vi "Compare local and remote personalities.vi"(8 "error in (no error)":errorcluster, 10 "DB personality":T1, 11 "roboRIO personality":T1) -> (0 "error out":errorcluster, 3 "Loaded Personality":T1)   [LabVIEW 2018, in "Personalities Tool.lvlib"]
doc: "This VI resolves conflicts between personalities in the roboRIO and in the local DB."
uses:
  Personalities Tool.lvlib
  Controls/Personality Type.ctl
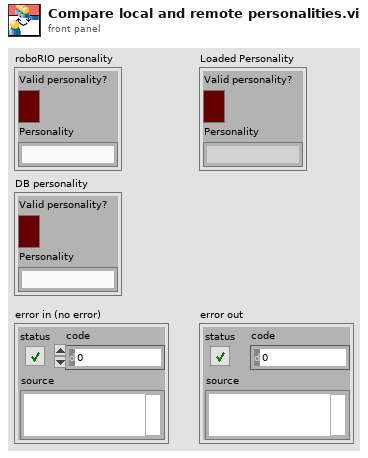
[diagram p1: front panel]
types:
  T1 = typedef "Personalities Tool.lvlib/Personality Type.ctl" = cluster{"Valid personality?":bool, "Personality":string}
  T2 = cluster{"Valid personality?":bool, "Personality":string}
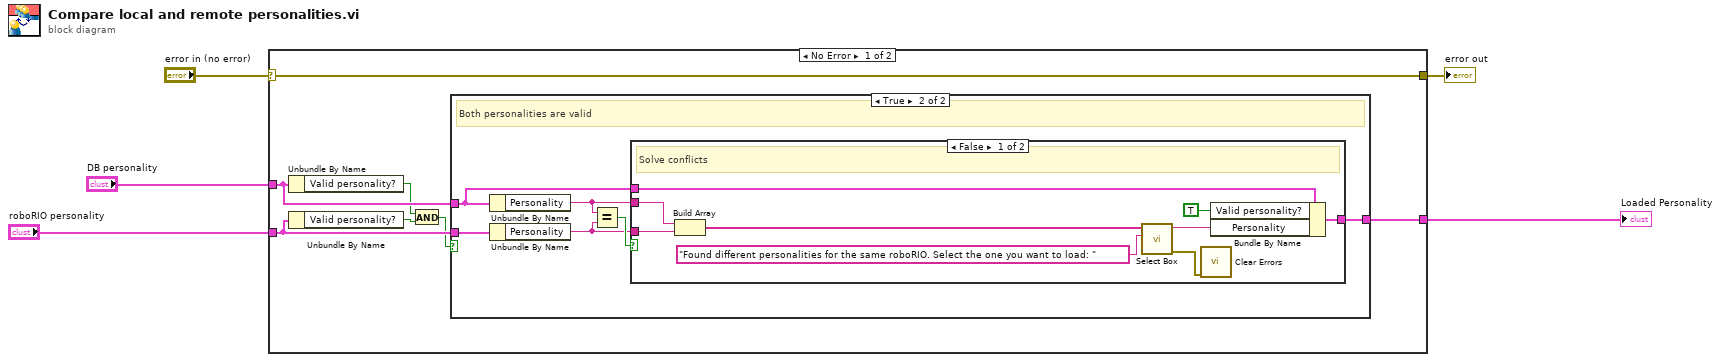
[diagram p0: block diagram]
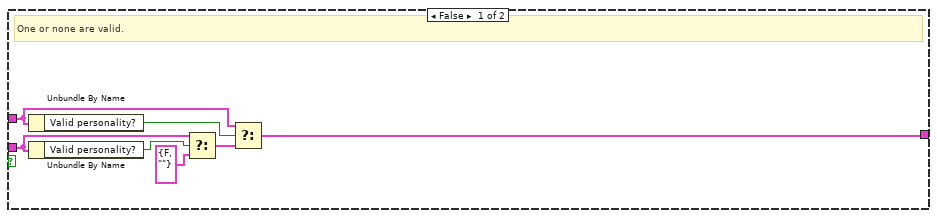
[diagram p2: hidden frame]
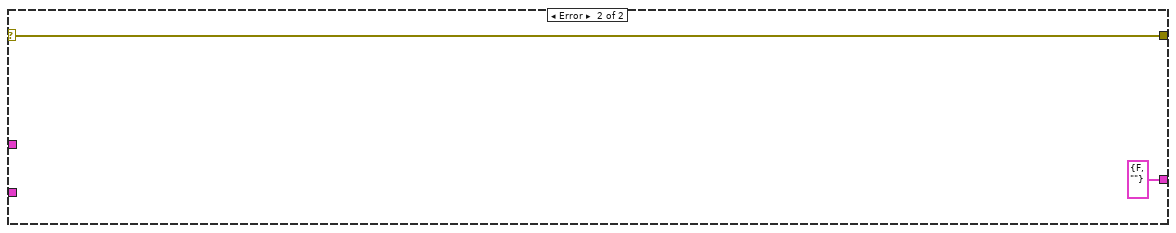
[diagram p4: hidden frame]
diagram:
  n1 = case shown="No Error" "error in (no error)" {
    selector: "error in (no error)" -> [w12 w37]
    tunnel: "roboRIO personality" -> [w11 _]
    tunnel: [w9 T2 {"Valid personality?"=FALSE, "Personality"=""} ("DB personality")] -> w2
    tunnel: [w12 w37] -> w3
    tunnel: "DB personality" -> [w10 _]
    frame No Error {
      n2 = Unbundle By Name(w10) -> ("Valid personality?"=w8:bool)
      n3 = Unbundle By Name(w11) -> ("Valid personality?"=w7:bool)
      n4 = And(x=w8, y=w7) -> (x .and. y?=w6:bool)
      n5 = case shown="True" w6 {
        tunnel: w11 -> [w18 w25]
        tunnel: w10 -> [w17 w22]
        tunnel: [w14 w23] -> w9
        frame False {
          # "One or none are valid."
          n6 = Unbundle By Name(w17) -> ("Valid personality?"=w16:bool)
          n7 = Unbundle By Name(w18) -> ("Valid personality?"=w19:bool)
          n8 = Select(t=w18, s=w19, f=T1 {"Valid personality?"=FALSE, "Personality"=""}) -> (s? t:f=w15:T1)
          n9 = Select(t=w17, s=w16, f=w15) -> (s? t:f=w14:T1)
        }
        frame True {
          # "Both personalities are valid"
          n10 = Unbundle By Name(w22) -> ("Personality"=w21:string)
          n11 = Unbundle By Name(w25) -> ("Personality"=w20:string)
          n12 = Equal?(x=w21, y=w20) -> (x = y?=w24:bool)
          n13 = case shown="False" w24 {
            tunnel: [w28 w35] -> w23
            tunnel: w22 -> [w30 w35]
            tunnel: w21 -> [w33 _]
            tunnel: w20 -> [w32 _]
            frame False {
              # "Solve conflicts"
              n14 = Build Array(w33, w32) -> (w31:string[])
              n15 = call "Select Box.vi"("UI message"="Found different personalities for the same roboRIO. Select the one you want to load: ", "Selections available"=w31) -> ("error out"=w26:errorcluster, "Selection"=w29:string)  [unwired: 8 in]
              n16 = call <vilib>:"Clear Errors.vi"("error in (no error)"=w26) -> ()  [unwired: 5 in, 2 out]
              n17 = Bundle By Name(cluster=w30, "Valid personality?"=TRUE, "Personality"=w29) -> (w28:T1)
            }
            frame True {
              # "Same personality"
            }
          }
        }
      }
    }
    frame Error {
    }
  }
  "error out" <- w3
  "Loaded Personality" <- w2
